vi "csm_lumikki_instron_status_poller.vi"   [LabVIEW 2009]
types:
  T1 = cluster{"Device ID":i32, "Device Name":string, "Device Type":i32}[]
  T2 = cluster{"Axis Information[0]":cluster{"Device ID":i32, "Device Name":string, "Device Type":i32}, "Axis Information[1]":cluster{"Device ID":i32, "Device Name":string, "Device Type":i32}, "Axis Information[2]":cluster{"Device ID":i32, "Device Name":string, "Device Type":i32}, "Axis Information[3]":cluster{"Device ID":i32, "Device Name":string, "Device Type":i32}, "Axis Information[4]":cluster{"Device ID":i32, "Device Name":string, "Device Type":i32}, "Axis Information[5]":cluster{"Device ID":i32, "Device Name":string, "Device Type":i32}, "Axis Information[6]":cluster{"Device ID":i32, "Device Name":string, "Device Type":i32}, "Axis Information[7]":cluster{"Device ID":i32, "Device Name":string, "Device Type":i32}, "Axis Information[8]":cluster{"Device ID":i32, "Device Name":string, "Device Type":i32}}
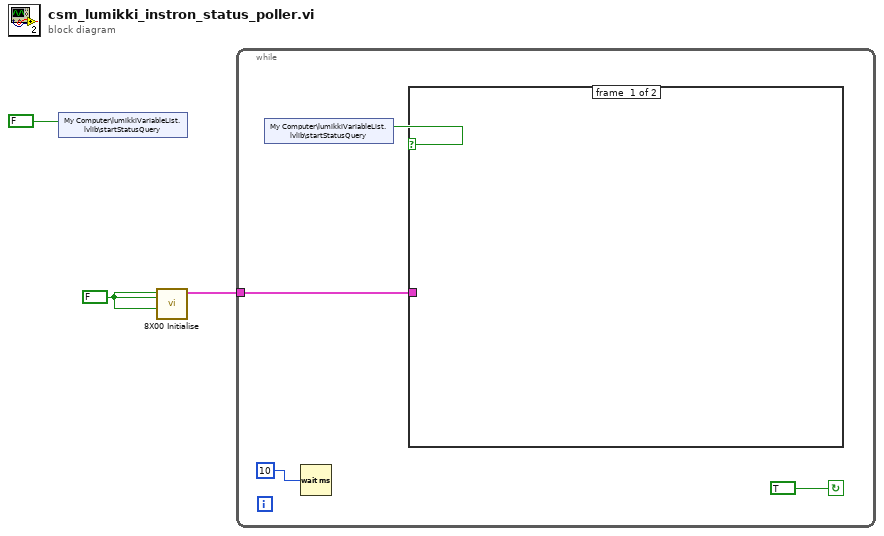
[diagram p0: block diagram]
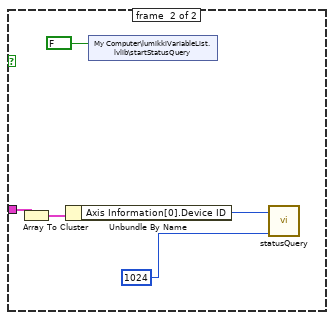
[diagram p2: hidden frame]
diagram:
  w3 = FALSE ("Create Console? (T)")
  n1 = shared-variable "My Computer\\lumikkiVariableList.lvlib\\startStatusQuery"(FALSE ("startStatusQuery")) -> ()  [unwired: 1 in, 1 out]
  n2 = call "8X00 Initialise.vi"("Reset?"=w3, "Create DVM? (T)"=w3, "Create Console? (T)"=w3) -> ("Axis Information"=w1:T1)  [unwired: 1 in, 3 out]
  n3 = while {
    tunnel: w1 -> [w4]
    stop <- TRUE continue-if-true
    n4 = shared-variable "My Computer\\lumikkiVariableList.lvlib\\startStatusQuery"() -> (w6:bool)  [unwired: 1 in, 1 out]
    n5 = Wait (ms)(milliseconds to wait=u32 10) -> ()  [unwired: 1 out]
    n6 = case shown="True" w6 {
      tunnel: w4 -> [_ w11]
      frame #0 {
      }
      frame #1 {
        n7 = Array To Cluster(array=w11) -> (cluster=w10:T2)
        n8 = Unbundle By Name(w10) -> ("Axis Information[0].Device ID"=w9:i32)
        n9 = shared-variable "My Computer\\lumikkiVariableList.lvlib\\startStatusQuery"(FALSE ("startRamp")) -> ()  [unwired: 1 in, 1 out]
        n10 = call "statusQuery.vi"("Reply size"=1024, "Device ID"=w9) -> ()  [unwired: 8 in, 2 out]
      }
    }
  }
